vi "Multidimensional Array.vi"() -> ()   [LabVIEW 2023]
panel:
  out "transposed Array":dbl[][](array[numeric])
  in  "Array":dbl[][](array[numeric])
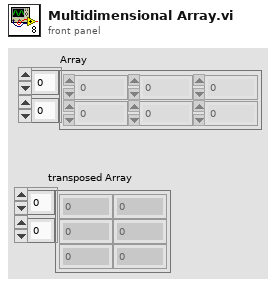
[diagram p1: front panel]
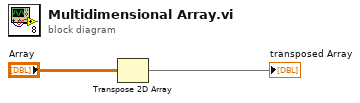
[diagram p0: block diagram]
diagram:
  n1 = Transpose 2D Array(2D array="Array") -> (transposed array=→"transposed Array":dbl[][])
